vi "user selectable OR constant.vi"(8 "Constant Path in":path, 10 "select source":enum32{"user selectable", "constant"}(ring), 11 "File Path in":path) -> (2 "appended path":path)   [LabVIEW 2011]
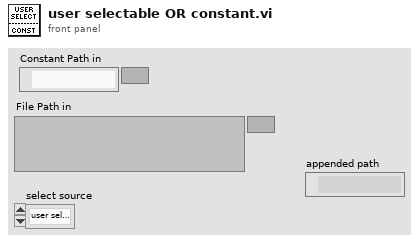
[diagram p1: front panel]
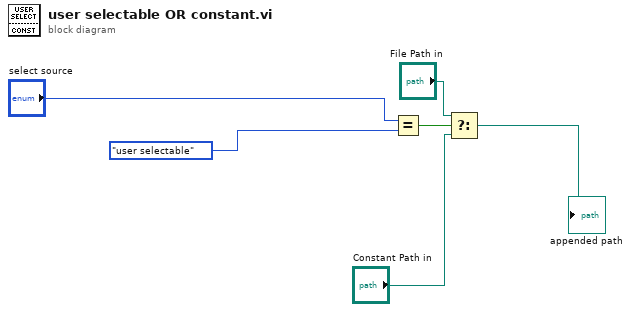
[diagram p0: block diagram]
diagram:
  n1 = Equal?(x="select source", y=enum32{"user selectable", "constant"}."user selectable") -> (x = y?=w4:bool)
  n2 = Select(t="File Path in", s=w4, f="Constant Path in") -> (s? t:f=→"appended path":path)
